vi "Get Variables.vi"(8 "error in":errorcluster, 10 "timed out?":bool, 11 "Data":T1) -> (0 "error out":errorcluster)   [LabVIEW 2026, in "Runtime Configuration Support Example Engine.lvlib"]
uses:
  HW Operations.ctl
  Runtime Configuration Support Example Engine.lvlib
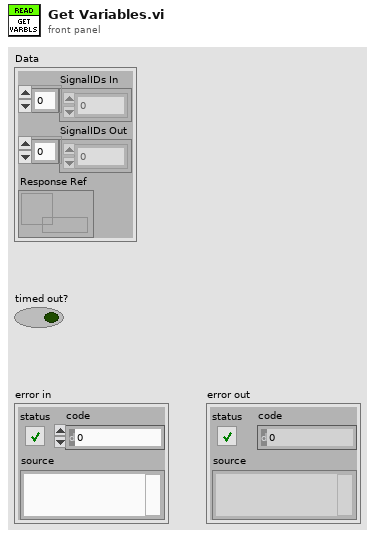
[diagram p1: front panel]
types:
  T1 = cluster{"SignalIDs In":i32[], "SignalIDs Out":i32[], "Response Ref":refnum<queue>}
  T2 = cluster{"SignalIDs In":i32[], "SignalIDs Out":i32[], "In Values":i32[], "Out Values":i32[], "Error":errorcluster}
  T3 = typedef "HW Operations.ctl" = enum16{"Initialize", "Set In Val", "Get In Val", "Set Block", "Set Out Val", "Get Out Val", "Get In Array", "Get Out Array"}
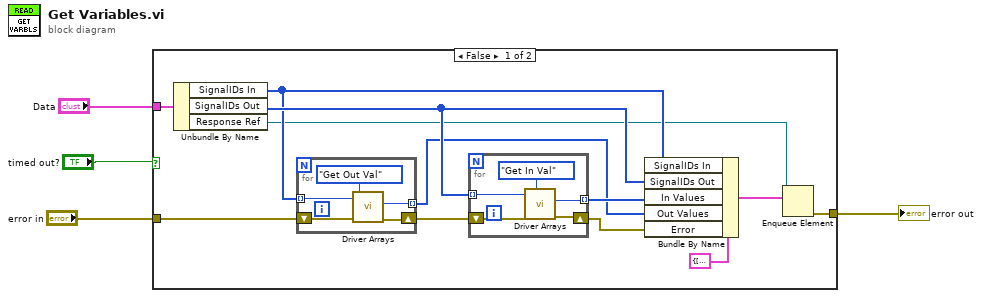
[diagram p0: block diagram]
diagram:
  n1 = case shown="False" "timed out?" {
    tunnel: "Data" -> [w12 _]
    tunnel: "error in" -> [w16 w27]
    tunnel: [w13 w27] -> w3
    frame False {
      n2 = Unbundle By Name(w12) -> ("SignalIDs In"=w8:i32[], "SignalIDs Out"=w10:i32[], "Response Ref"=w5:refnum<queue>)
      n3 = for {
        tunnel: w8 -> [w19] mode=indexing
        tunnel: [w17] -> w7 mode=indexing
        shift-right: [w20] -> w15
        shift-left: w16 -> [w21]
        n4 = call "Driver Arrays.vi"("error in"=w21, "Index"=w19, "Curr Operation"=HW_Operations."Get Out Val") -> ("error out"=w20:errorcluster, "Value"=w17:i32)  [unwired: 5 in, 2 out]
      }
      n5 = for {
        tunnel: w10 -> [w24] mode=indexing
        tunnel: [w22] -> w11 mode=indexing
        shift-right: [w25] -> w14
        shift-left: w15 -> [w26]
        n6 = call "Driver Arrays.vi"("error in"=w26, "Index"=w24, "Curr Operation"=HW_Operations."Get In Val") -> ("error out"=w25:errorcluster, "Value"=w22:i32)  [unwired: 5 in, 2 out]
      }
      n7 = Bundle By Name(cluster=T2 {"SignalIDs In"=[], "SignalIDs Out"=[], "In Values"=[], "Out Values"=[], "Error"={"status"=FALSE, "code"=0, "source"=""}}, "SignalIDs In"=w8, "SignalIDs Out"=w10, "In Values"=w11, "Out Values"=w7, "Error"=w14) -> (w6:T2)
      n8 = Enqueue Element(queue=w5, element=w6) -> (error out=w13:errorcluster)  [unwired: 2 in, 2 out]
    }
    frame True {
    }
  }
  "error out" <- w3
